vi "Write Alazar DAQ Parameters.vi"(8 "error in (no error)":errorcluster, 10 "Device":T1={"Record"={"Count"=0, "Presize"=0, "Length"=0}, "Clock"={"ClckSource"=enum."Internal", "ClckRate"=0, "ClckEdge"=0, "Decimation"=0}, "Input A"={"Coupling"=enum."DC", "Range"=12, "Impedance"=enum."1M ohms", "Bandwidth"=enum."Full Bandwidth"}, "Input B"={"Coupling"=enum."DC", "Range"=12, "Impedance"=enum."1M ohms", "Bandwidth"=enum."Full Bandwidth"}, "Trigger"={"TrigOperation"=enum."Only X", "Timeout (s)"=-1.0, "Trig. Delay"=0, "Engine X"={"Source"=enum."Chan_A", "Slope"=enum."Positive", "Level"=0}, "Engine Y"={"Source"=enum."Chan_A", "Slope"=enum."Positive", "Level"=0}, "ExtTrigControl"={"Coupling"=enum."AC", "Range"=enum."1 V"}}} {"Clock"."ClckEdge" items=["Rising", "Falling"]; "Clock"."ClckRate" items=["1 kS/s", "2 kS/s", "5 kS/s", "10 kS/s", "20 kS/s", "50 kS/s", "100 kS/s", "200 kS/s", "500 kS/s", "1 MS/s", "2 MS/s", "5 MS/s", "10 MS/s", "20 MS/s", "25 MS/s", "50 MS/s", "100 MS/s", "125 MS/s", "200 MS/s", "250 MS/s", "500 MS/s", "1 GS/s"]; "Input B"."Range" items=["20mv", "40mV", "50mV", "80mV", "100mV", "200mV", "400mV", "500mV", "800mV", "1 V", "2 V", "4 V", "5 V", "8 V", "10 V", "20 V"]; "Trigger"."Timeout (s)" format="%.2f"; "Input A"."Range" items=["20mv", "40mV", "50mV", "80mV", "100mV", "200mV", "400mV", "500mV", "800mV", "1 V", "2 V", "4 V", "5 V", "8 V", "10 V", "20 V"]}, 11 "ATS660 Class in":refnum<class "ATS660 Class.lvclass">) -> (0 "error out":errorcluster, 3 "ATS660 Class out":refnum<class "ATS660 Class.lvclass">)   [LabVIEW 2015, in "ATS660 Class.lvclass"]
uses:
  ATS660 Class.lvclass
  ATS-VI/ATS_ctl/ATS_Global.ctl
  ATS-VI/ATS_ctl/Record.ctl
  ATS-VI/ATS_ctl/Clock.ctl
  ATS-VI/ATS_ctl/ClockSource.ctl
  ATS-VI/ATS_ctl/ClockRate.ctl
  ATS-VI/ATS_ctl/ClockEdge.ctl
  ATS-VI/ATS_ctl/InputCtrl.ctl
  ATS-VI/ATS_ctl/Coupling.ctl
  ATS-VI/ATS_ctl/Range.ctl
  ATS-VI/ATS_ctl/Impedance.ctl
  ATS-VI/ATS_ctl/Bandwidth.ctl
  ATS-VI/ATS_ctl/Trigger.ctl
  ATS-VI/ATS_ctl/TriggerOperation.ctl
  ATS-VI/ATS_ctl/TriggerEngine.ctl
  ATS-VI/ATS_ctl/ExtTrigger.ctl
  ATS-VI/ATS_ctl/ExtTrigRange.ctl
  ATS660 Class.lvclass/ATS660 Class.ctl
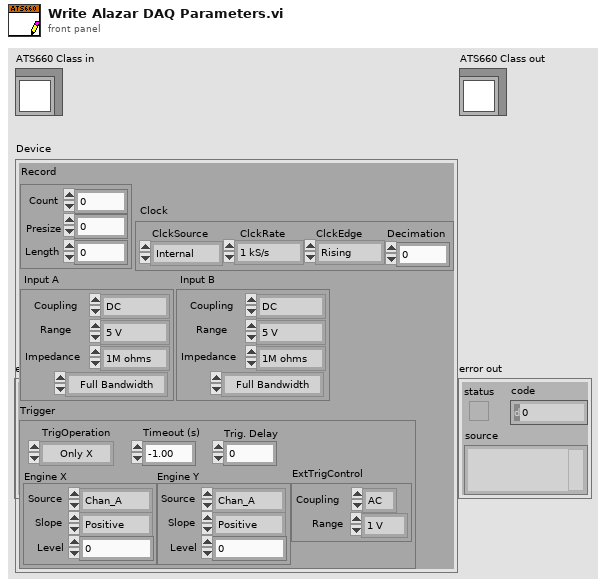
[diagram p1: front panel]
types:
  T1 = typedef "ATS_Global.ctl" = cluster{"Record":T2, "Clock":T3, "Input A":T7, "Input B":T7, "Trigger":T12}
  T2 = typedef "Record.ctl" = cluster{"Count":u32, "Presize":u32, "Length":u32}
  T3 = typedef "Clock.ctl" = cluster{"ClckSource":T4, "ClckRate":T5, "ClckEdge":T6, "Decimation":u32}
  T4 = typedef "ClockSource.ctl" = enum16{"Internal", "External", "Medium Ext.", "Slow Ext.", "Ext. AC", "Ext. DC", "Ext. (PLL)"}
  T5 = typedef "ClockRate.ctl" = u32
  T6 = typedef "ClockEdge.ctl" = u16
  T7 = typedef "InputCtrl.ctl" = cluster{"Coupling":T8, "Range":T9, "Impedance":T10, "Bandwidth":T11}
  T8 = typedef "Coupling.ctl" = enum16{"AC", "DC"}
  T9 = typedef "Range.ctl" = u32
  T10 = typedef "Impedance.ctl" = enum16{"1M ohms", "50 ohms"}
  T11 = typedef "Bandwidth.ctl" = enum16{"Full Bandwidth", "Reduce Bandwidth"}
  T12 = typedef "Trigger.ctl" = cluster{"TrigOperation":T13, "Timeout (s)":dbl, "Trig. Delay":u32, "Engine X":T14, "Engine Y":T14, "ExtTrigControl":T15}
  T13 = typedef "TriggerOperation.ctl" = enum16{"Only X", "Only Y", "X or Y", "X and Y", "X xor Y", "X and not Y", "not X and Y"}
  T14 = typedef "TriggerEngine.ctl" = cluster{"Source":enum32{"Chan_A", "Chan_B", "External", "Disable"}, "Slope":enum32{"Positive", "Negative"}, "Level":u32}
  T15 = typedef "ExtTrigger.ctl" = cluster{"Coupling":T8, "Range":T16}
  T16 = typedef "ExtTrigRange.ctl" = enum16{"1 V", "5 V", "TTL"}
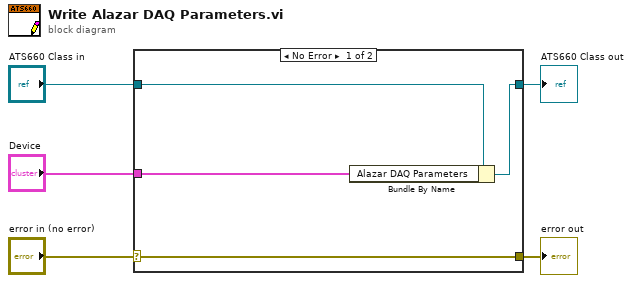
[diagram p0: block diagram]
diagram:
  n1 = case shown="No Error" "error in (no error)" {
    selector: "error in (no error)" -> [w9 w10]
    tunnel: [w9 w10] -> w4
    tunnel: [w7 w11] -> w2
    tunnel: "ATS660 Class in" -> [w8 w11]
    tunnel: "Device" -> [w6 _]
    frame No Error {
      n2 = Bundle By Name(cluster=w8, "Alazar DAQ Parameters"=w6) -> (w7:refnum<class "ATS660 Class.lvclass">)
    }
    frame Error {
    }
  }
  "error out" <- w4
  "ATS660 Class out" <- w2
